vi "Set X Maximum.vi"(9 "Graph Reference Cluster":T1, 11 "Display Size":T2(ring)) -> ()   [LabVIEW 2014]
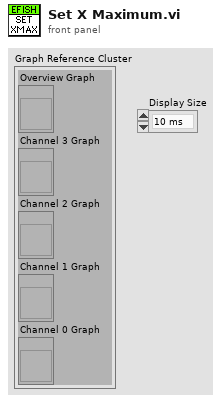
[diagram p1: front panel]
types:
  T1 = cluster{"Overview Graph":refnum<vi>, "Channel 3 Graph":refnum<vi>, "Channel 2 Graph":refnum<vi>, "Channel 1 Graph":refnum<vi>, "Channel 0 Graph":refnum<vi>}
  T2 = enum16{"10 ms", "100 ms", "1 Second", "10 sec", "30 sec"}
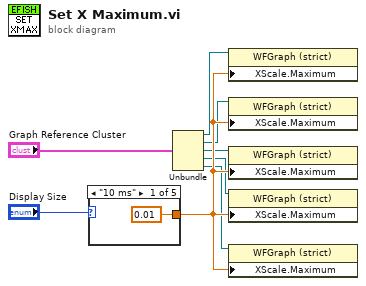
[diagram p0: block diagram]
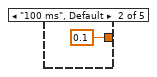
[diagram p2: hidden frame]
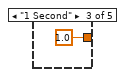
[diagram p3: hidden frame]
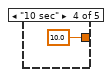
[diagram p4: hidden frame]
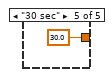
[diagram p5: hidden frame]
diagram:
  n1 = case shown="\"10 ms\"" "Display Size" {
    tunnel: [0.01 0.1 1.0 10.0 30.0] -> w8
    frame "10 ms" {
    }
    frame "100 ms", Default {
    }
    frame "1 Second" {
    }
    frame "10 sec" {
    }
    frame "30 sec" {
    }
  }
  n2 = Unbundle("Graph Reference Cluster") -> ("Overview Graph"=w6:refnum<vi>, "Channel 3 Graph"=w5:refnum<vi>, "Channel 2 Graph"=w4:refnum<vi>, "Channel 1 Graph"=w3:refnum<vi>, "Channel 0 Graph"=w2:refnum<vi>)
  n3 = property on="Property Node" class="WFGraph (strict)"(reference=w6, "XScale.Maximum"=w8) -> ()  [unwired: 1 in, 2 out]
  n4 = property on="Property Node" class="WFGraph (strict)"(reference=w5, "XScale.Maximum"=w8) -> ()  [unwired: 1 in, 2 out]
  n5 = property on="Property Node" class="WFGraph (strict)"(reference=w4, "XScale.Maximum"=w8) -> ()  [unwired: 1 in, 2 out]
  n6 = property on="Property Node" class="WFGraph (strict)"(reference=w3, "XScale.Maximum"=w8) -> ()  [unwired: 1 in, 2 out]
  n7 = property on="Property Node" class="WFGraph (strict)"(reference=w2, "XScale.Maximum"=w8) -> ()  [unwired: 1 in, 2 out]
